vi "SubVI_Predict_on_Window.vi"(1 "Protocol waiting period":dbl, 4 "Minimum Imagine Limit":dbl, 6 "Covariance Matrix":dbl[][](array[numeric]), 7 "Time Window":dbl[](array[numeric]), 8 "error in (no error)":errorcluster, 9 "GO Epoch Means":dbl[](array[numeric]), 10 "Hyperparameters":T1, 11 "Spatial Mean In":T2) -> (0 "error out":errorcluster)   [LabVIEW 2020]
uses:
  <extravilib>/ChannelInstances/Stream-a[.,.](dbl)/)Channel.ctl
  <vilib>/Analysis/baseanly.llb/Mean (DBL).vi
  <extravilib>/ChannelInstances/Stream-a[.,.](dbl)/EndpointRead.vi
  Global 1.vi
  <extravilib>/ChannelInstances/Stream-a[.,.](dbl)/)Channel.vi
  <resource>/ChannelSupport/_ChannelSupport/WaitIfNeeded.vi
  <extravilib>/ChannelInstances/Stream-a[.,.](dbl).lvlib
  <vilib>/Analysis/NI_AALBase.lvlib
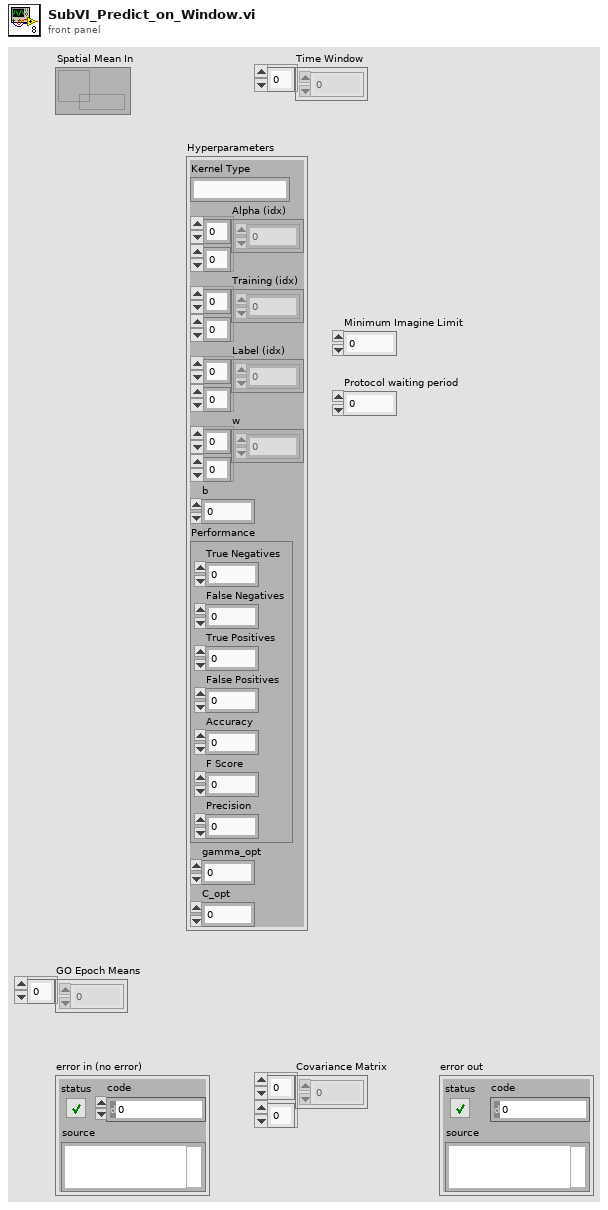
[diagram p1: front panel]
types:
  T1 = cluster{"Kernel Type":string, "Alpha (idx)":dbl[][], "Training (idx)":dbl[][], "Label (idx)":dbl[][], "w":dbl[][], "b":dbl, "Performance":cluster{"True Negatives":i32, "False Negatives":i32, "True Positives":i32, "False Positives":i32, "Accuracy":dbl, "F Score":dbl, "Precision":dbl}, "gamma_opt":dbl, "C_opt":dbl}
  T2 = typedef "Stream-a[.,.](dbl).lvlib/)Channel.ctl" = refnum<queue>
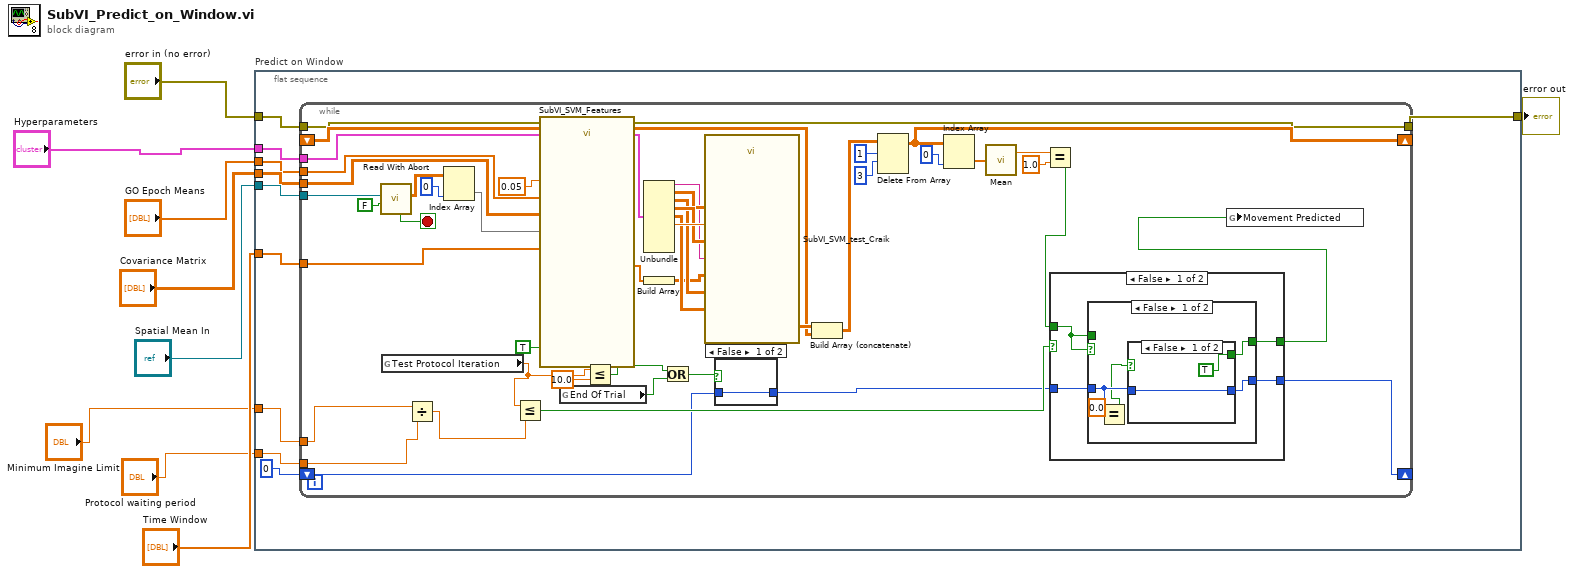
[diagram p0: block diagram]
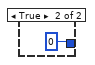
[diagram p2: hidden frame]
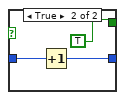
[diagram p3: hidden frame]
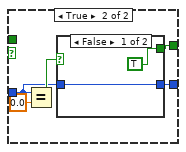
[diagram p4: hidden frame]
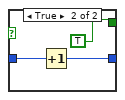
[diagram p5: hidden frame]
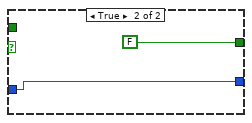
[diagram p6: hidden frame]
diagram:
  n1 = flat-sequence "Predict on Window" {
    tunnel: "Time Window" -> [w19]
    tunnel: "Spatial Mean In" -> [w18]
    tunnel: "Covariance Matrix" -> [w17]
    tunnel: "GO Epoch Means" -> [w16]
    tunnel: "Hyperparameters" -> [w15]
    tunnel: "error in (no error)" -> [w14]
    tunnel: [w13] -> w8
    tunnel: "Minimum Imagine Limit" -> [w12]
    tunnel: "Protocol waiting period" -> [w11]
    frame #0 {
      n2 = while {
        tunnel: w18 -> [w64]
        tunnel: w16 -> [w62]
        tunnel: w17 -> [w61]
        tunnel: w19 -> [w60]
        tunnel: w15 -> [w48]
        shift-right: [w41] -> _
        shift-left: _ -> [w45]
        tunnel: w14 -> [w35]
        tunnel: [w35] -> w13
        tunnel: w12 -> [w32]
        tunnel: w11 -> [w31]
        shift-right: [w28] -> _
        shift-left: 0 -> [w23]
        stop <- w36 stop-if-true
        n3 = call <extravilib>:"Read With Abort.vi"("abort"=FALSE, "channel"=w64) -> ("element"=w59:dbl[][], "aborted?"=w36:bool)  [unwired: 4 in, 4 out]
        n4 = global read "Global 1.vi" "Test Protocol Iteration"() -> (w27:dbl)
        n5 = Divide(x=w32, y=w31) -> (x/y=w30:dbl)
        n6 = Index Array(array=w59, index (col)=0 ("index (row)")) -> (element=w56:dbl[])  [unwired: 1 in]
        n7 = Less Or Equal?(x=w27, y=w30) -> (x <= y?=w29:bool)
        n8 = call "SubVI_SVM_Features.vi"("Sigma"=w61, "MU"=w62, "Scale?"=TRUE, "dt"=0.05, "window_time"=w60, "Sliding_window"=w56) -> ("Features_array"=w58:dbl[])  [unwired: 1 in, 4 out]
        n9 = global read "Global 1.vi" "End Of Trial"() -> (w24:bool)
        n10 = Less Or Equal?(x=w27, y=10.0) -> (x <= y?=w25:bool)
        n11 = Unbundle(w48) -> ("Kernel Type"=w49:string, "Alpha (idx)"=w50:dbl[][], "Training (idx)"=w51:dbl[][], "Label (idx)"=w52:dbl[][], "w"=w53:dbl[][], "b"=w54:dbl)  [unwired: 3 out]
        n12 = Build Array(w58) -> (w47:dbl[][])
        n13 = Or(x=w25, y=w24) -> (x .or. y?=w21:bool)
        n14 = call "SubVI_SVM_test_Craik.vi"("Alpha (idx)"=w50, "Testing Data"=w47, "Label (idx)"=w52, "training (idx)"=w51, "Linear or Gaussian"=w49, "b"=w54, "w"=w53) -> ("Prediction"=w46:dbl[][])  [unwired: 4 in]
        n15 = case shown="False" w21 {
          tunnel: w23 -> [w65 _]
          tunnel: [w65 0] -> w22
          frame False {
          }
          frame True {
          }
        }
        n16 = Build Array (concatenate)(w46, w45) -> (w44:dbl[][])
        n17 = Delete From Array(array=w44, length=1, index (row)=3) -> (array with subset deleted=w41:dbl[][])  [unwired: 1 in, 1 out]
        n18 = Index Array(array=w41, index (col)=0 ("disabled index (col)")) -> (element=w40:dbl[])  [unwired: 1 in]
        n19 = call-poly <vilib>:"Mean.vi"("X"=w40) -> ("mean"=w38:dbl)  [unwired: 1 out]
        n20 = Equal?(x=w38, y=1.0) -> (x = y?=w33:bool)
        n21 = case shown="False" w29 {
          tunnel: [w70 FALSE ("Movement Predicted")] -> w34
          tunnel: w33 -> [w69 _]
          tunnel: w22 -> [w68 w91]
          tunnel: [w67 w91] -> w28
          frame False {
            n22 = case shown="False" w69 {
              tunnel: [w73 w81] -> w70
              tunnel: w69 -> [_ _]
              tunnel: w68 -> [w74 w83]
              tunnel: [w72 w82] -> w67
              frame False {
                n23 = Equal?(x=w74, y=0.0) -> (x = y?=w71:bool)
                n24 = case shown="False" w71 {
                  tunnel: w74 -> [w77 w80]
                  tunnel: [w77 w79] -> w72
                  tunnel: [TRUE TRUE] -> w73
                  frame False {
                  }
                  frame True {
                    n25 = Increment(x=w80) -> (x+1=w79:i32)
                  }
                }
              }
              frame True {
                n26 = Equal?(x=w83, y=0.0) -> (x = y?=w84:bool)
                n27 = case shown="False" w84 {
                  tunnel: w83 -> [w87 w90]
                  tunnel: [w87 w89] -> w82
                  tunnel: [TRUE TRUE] -> w81
                  frame False {
                  }
                  frame True {
                    n28 = Increment(x=w90) -> (x+1=w89:i32)
                  }
                }
              }
            }
          }
          frame True {
          }
        }
        n29 = global write "Global 1.vi" "Movement Predicted"(w34) -> ()
      }
    }
  }
  "error out" <- w8
